vi "Randomize Numerical Array.vi"(11 "Array":dbl[](array[numeric])=[0.0, 1.0, 2.0, 3.0, 4.0, 5.0, 6.0, 7.0, 8.0, 9.0]) -> (3 "Randomized Array":dbl[](array[numeric]))   [LabVIEW 2021]
doc: "Demonstrates how to randomize the order of an array"
panel:
  # "Overview: Demonstrates how to randomize the order of an array\nRequirements: LabVIEW 2012 Base Development System (or compatible)\n\nInstructions: \n1. (Optional) Change array or use this VI as an subVI\n2. Run the VI"
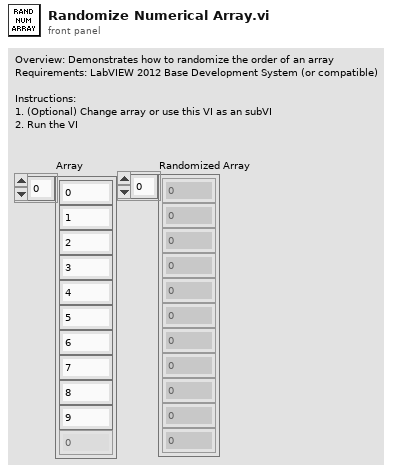
[diagram p1: front panel]
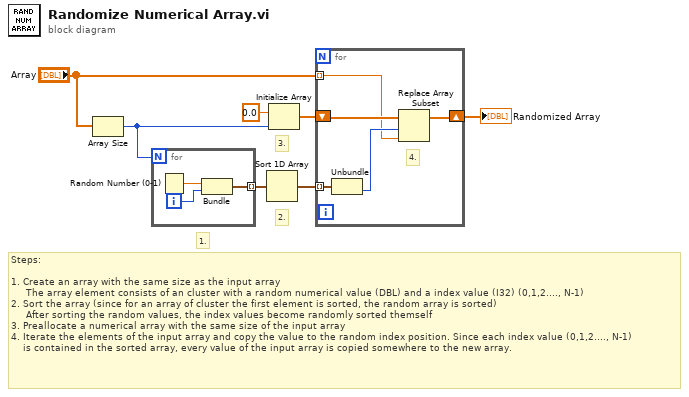
[diagram p0: block diagram]
diagram:
  # "3."
  # "2."
  # "1."
  # "Steps:\n\n1. Create an array with the same size as the input array\n     The array element consists of an cluster with a random numerical value (DBL) and a index value (I32) (0,1,2...., N-1)\n2. Sort the array (since for an array of cluster the first element is sorted, the random array is sorted)\n     After sorting the random values, the index values become randomly sorted themself\n3. Preallocate a numerical array with the same size of the input array\n4. Iterate the elements of the input array and copy the value to the random index position. Since each index value (0,1,2...., N-1)\n    is contained in the sorted array, every value of the input array is copied somewhere to the new array."
  n1 = Array Size(array="Array") -> (size(s)=w1:i32)
  n2 = for {
    N: w1 -> [_]
    tunnel: [w9] -> w2 mode=indexing
    i -> [w10]
    n3 = Random Number (0-1)() -> (number: 0 to 1=w8:dbl)
    n4 = Bundle("number: 0 to 1"=w8, w10) -> (w9:cluster{"number: 0 to 1":dbl, i32})  [unwired: 1 in]
  }
  n5 = Sort 1D Array(array=w2) -> (sorted array=w3:cluster{"number: 0 to 1":dbl, i32}[])
  n6 = Initialize Array(0.0 ("element"), w1) -> (w5:dbl[])
  n7 = for {
    tunnel: w3 -> [w15] mode=indexing
    shift-right: [w13] -> w7
    shift-left: w5 -> [w14]
    tunnel: "Array" -> [w11] mode=indexing
    # "4."
    n8 = Unbundle(w15) -> (w12:i32)  [unwired: 1 out]
    n9 = Replace Array Subset(array=w14, new element=w11, index=w12) -> (w13:dbl[])
  }
  "Randomized Array" <- w7
